vi "ADAM_paralelo.vi"() -> ()   [LabVIEW 2019]
uses:
  <vilib>/Instr/_visa.llb/VISA Configure Serial Port (Instr).vi
  padrao_ADAM_SAIDA.ctl
  padrao_ADAM_ENTRADA.ctl
panel:
  in  "ADAM_ENTRADA":T1
  in  "VISA resource name":refnum<visa-resource-name>
  in  "ADAM_SAIDA":T2
  in  "ESC":bool
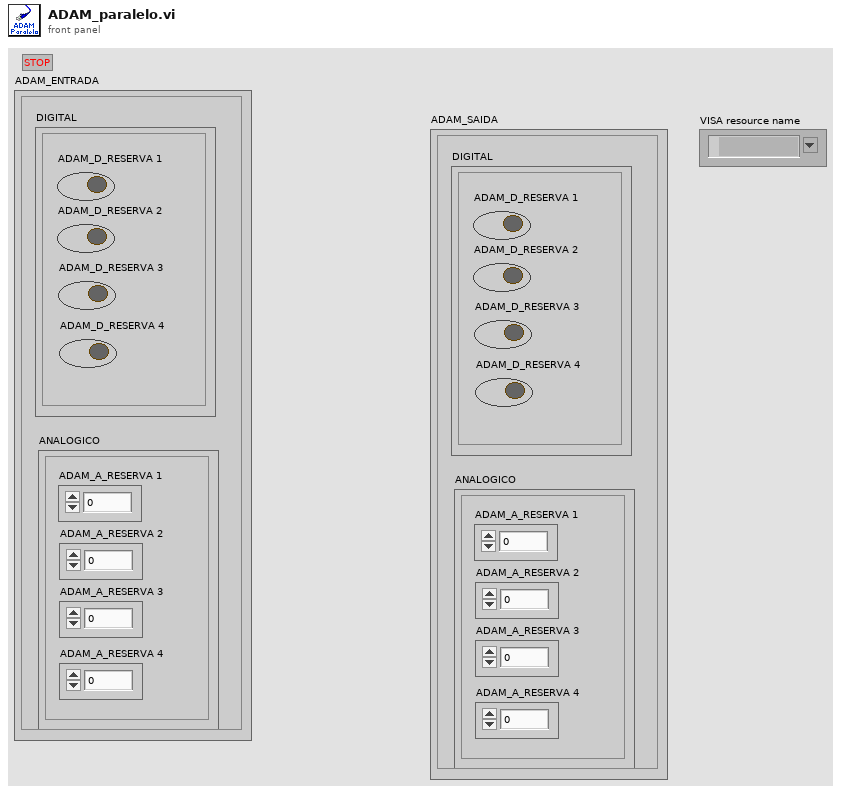
[diagram p1: front panel]
types:
  T1 = typedef "padrao_ADAM_ENTRADA.ctl" = cluster{"DIGITAL":cluster{"ADAM_D_RESERVA 1":bool, "ADAM_D_RESERVA 2":bool, "ADAM_D_RESERVA 3":bool, "ADAM_D_RESERVA 4":bool}, "ANALOGICO":cluster{"ADAM_A_RESERVA 1":dbl, "ADAM_A_RESERVA 2":dbl, "ADAM_A_RESERVA 3":dbl, "ADAM_A_RESERVA 4":dbl}}
  T2 = typedef "padrao_ADAM_SAIDA.ctl" = cluster{"DIGITAL":cluster{"ADAM_D_RESERVA 1":bool, "ADAM_D_RESERVA 2":bool, "ADAM_D_RESERVA 3":bool, "ADAM_D_RESERVA 4":bool}, "ANALOGICO":cluster{"ADAM_A_RESERVA 1":dbl, "ADAM_A_RESERVA 2":dbl, "ADAM_A_RESERVA 3":dbl, "ADAM_A_RESERVA 4":dbl}}
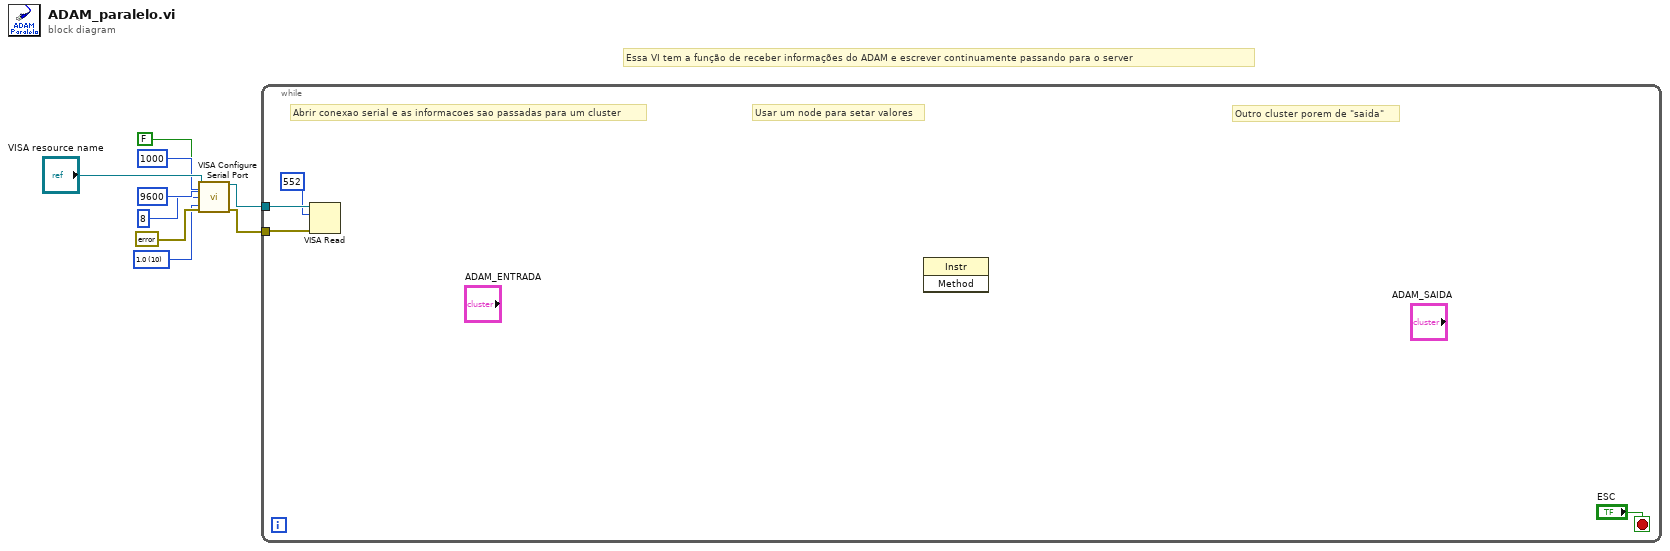
[diagram p0: block diagram]
diagram:
  w1 = u16 10 items=["1.0"=10, "1.5"=15, "2.0"=20] ("stop bits (10: 1 bit)")
  # "Essa VI tem a função de receber informações do ADAM e escrever continuamente passando para o server"
  n1 = call-poly "VISA Configure Serial Port"("VISA resource name"="VISA resource name", "timeout (10sec)"=u32 1000, "Enable Termination\nChar (T)"=FALSE ("Enable Termination\nChar (T)"), "baud rate (9600)"=u32 9600, "data bits (8)"=u16 8, "error in (no error)"=errorcluster {"status"=FALSE, "code"=0, "source"=""}, "stop bits (10: 1 bit)"=w1) -> ("VISA resource name out"=w6:refnum<visa-resource-name>, "error out"=w9:errorcluster)  [unwired: 7 in]
  n2 = while {
    tunnel: w9 -> [w11]
    tunnel: w6 -> [w12]
    stop <- "ESC" stop-if-true
    # "Outro cluster porem de \"saida\""
    # "Usar um node para setar valores"
    # "Abrir conexao serial e as informacoes sao passadas para um cluster"
    n3 = VISA Read(VISA resource name=w12, byte count=u32 552, error in (no error)=w11) -> ()  [unwired: 4 out]
    n4 = invoke class="Instr" method=#-1() -> ()  [unwired: 3 in, 3 out]
  }
